vi "fgv_imu_data.vi"(7 "cmd":T1, 8 "error in":errorcluster, 11 "IMD data":T2) -> (0 "error out":errorcluster, 1 "heading":dbl, 2 "ang":dbl[](array[numeric]), 3 "IMD data out":T2)   [LabVIEW 2019]
uses:
  Ctrl/cmd_imu.ctl
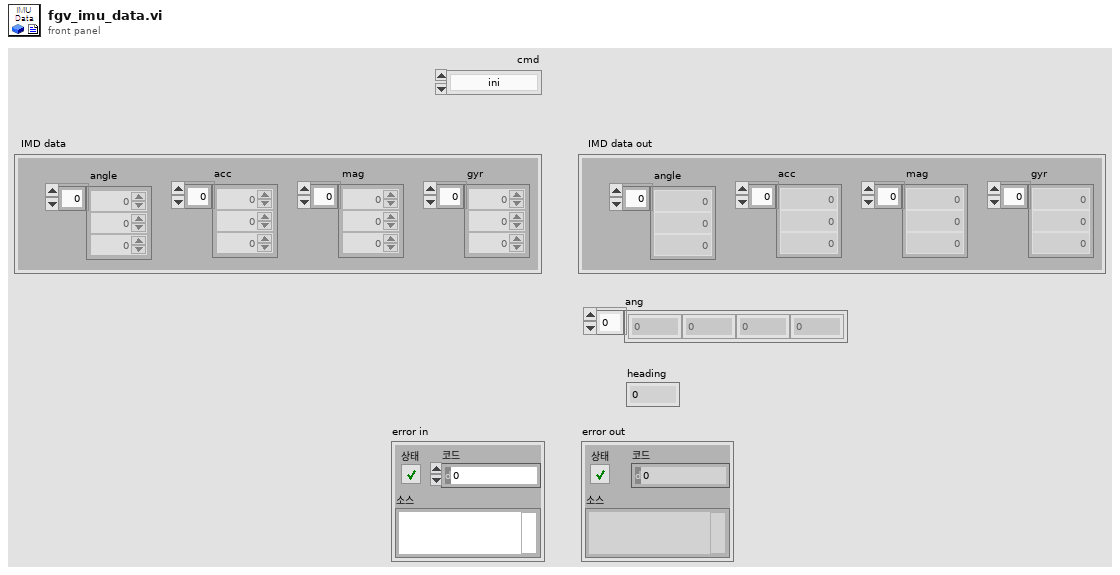
[diagram p1: front panel]
types:
  T1 = typedef "cmd_imu.ctl" = enum16{"ini", "write", "read"}
  T2 = cluster{"angle":dbl[], "acc":dbl[], "mag":dbl[], "gyr":dbl[]}
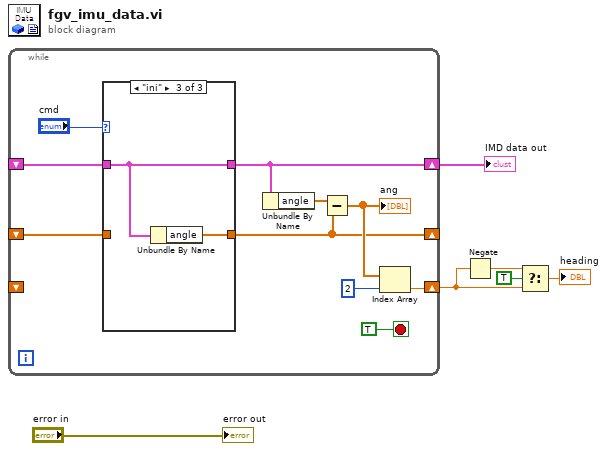
[diagram p0: block diagram]
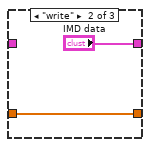
[diagram p3: hidden frame]
diagram:
  n1 = while {
    shift-right: [w15] -> w5
    shift-left: _ -> [w14]
    shift-right: [w9] -> _
    shift-left: _ -> [w12]
    shift-right: [w7] -> w3
    shift-left: _ -> [_]
    stop <- TRUE stop-if-true
    n2 = case shown="\"ini\"" "cmd" {
      tunnel: [w18 "IMD data" w22] -> w15
      tunnel: w14 -> [w18 _ w22]
      tunnel: [w17 w19 w21] -> w9
      tunnel: w12 -> [w17 w19 _]
      frame "read", Default {
      }
      frame "write" {
      }
      frame "ini" {
        n3 = Unbundle By Name(w22) -> ("angle"=w21:dbl[])
      }
    }
    n4 = Unbundle By Name(w15) -> ("angle"=w11:dbl[])
    n5 = Subtract(x=w11, y=w9) -> (x-y=w10:dbl[])
    "ang" <- w10
    n6 = Index Array(array=w10, index=2 ("인덱스")) -> (element=w7:dbl)
  }
  "IMD data out" <- w5
  n7 = Negate(x=w3) -> (-x=w4:dbl)
  n8 = Select(t=w4, s=TRUE, f=w3) -> (s? t:f=→"heading":dbl)
  "error out" <- "error in"
